vi "get_done_flag.vi"(8 "error in (no error)":errorcluster, 11 "GenericSweep in":refnum<class "GenericSweep.lvclass">) -> (0 "error out":errorcluster, 2 "sweep done?":bool, 3 "GenericSweep out":refnum<class "GenericSweep.lvclass">)   [LabVIEW 2010, in "GenericSweep.lvclass"]
uses:
  GenericSweep.lvclass
  GenericSweep.lvclass/GenericSweep.ctl
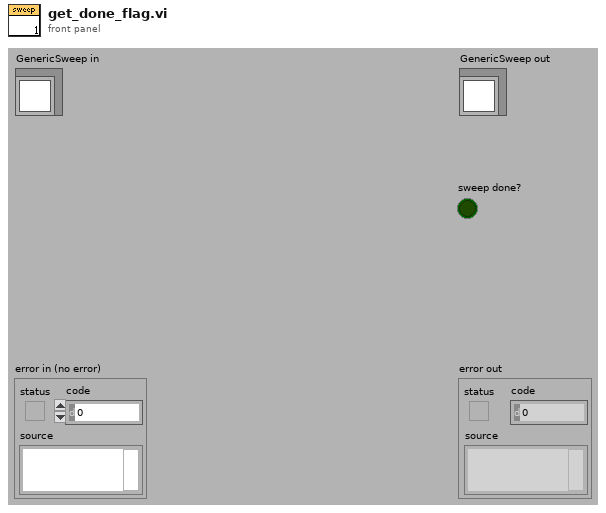
[diagram p1: front panel]
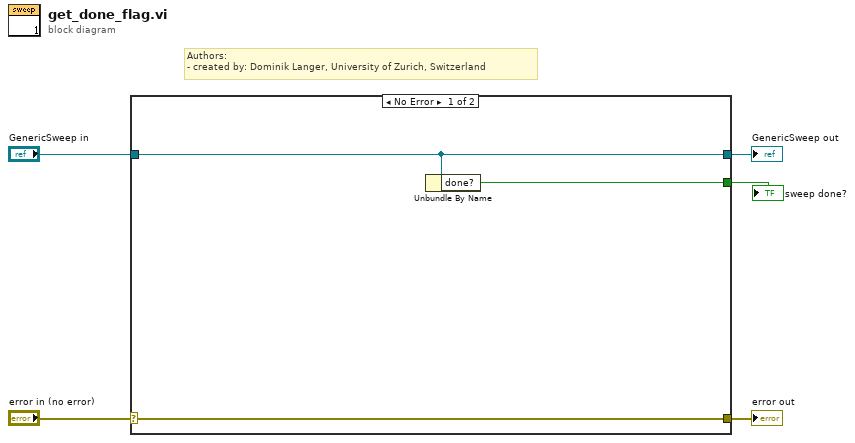
[diagram p0: block diagram]
diagram:
  # "Authors: \n- created by: Dominik Langer, University of Zurich, Switzerland"
  n1 = case shown="No Error" "error in (no error)" {
    selector: "error in (no error)" -> [w8 w10]
    tunnel: [w8 w10] -> w4
    tunnel: [w7 w9] -> w2
    tunnel: "GenericSweep in" -> [w7 w9]
    tunnel: [w6 _] -> w1
    frame No Error {
      n2 = Unbundle By Name(w7) -> ("done?"=w6:bool)
    }
    frame Error {
    }
  }
  "error out" <- w4
  "GenericSweep out" <- w2
  "sweep done?" <- w1
